vi "LJT4_end.vi"(8 "error in":errorcluster, 11 "Handle Out":i32) -> (3 "String":string)   [LabVIEW 2019]
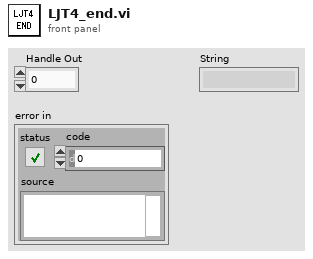
[diagram p1: front panel]
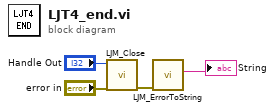
[diagram p0: block diagram]
diagram:
  n1 = call "LJM_Close.vi"("error in"="error in", "Handle"="Handle Out") -> ("error out"=w3:errorcluster)  [unwired: 9 in]
  n2 = call "LJM_ErrorToString.vi"("error in"=w3) -> ("String"=→"String":string)  [unwired: 10 in]
